vi "Configure Regulation Speed.vi"(8 "error in (no error)":errorcluster, 10 "Regulation Speed (1: Medium)":u16(ring)=1 items=["Slow", "Medium", "Fast"], 11 "VISA resource name":refnum<visa-resource-name>) -> (0 "error out":errorcluster, 3 "VISA resource name out":refnum<visa-resource-name>)   [LabVIEW 2017, in "HH PLI Series.lvlib"]
doc: "Sets the regulation speed of the instrument controller."
uses:
  HH PLI Series.lvlib
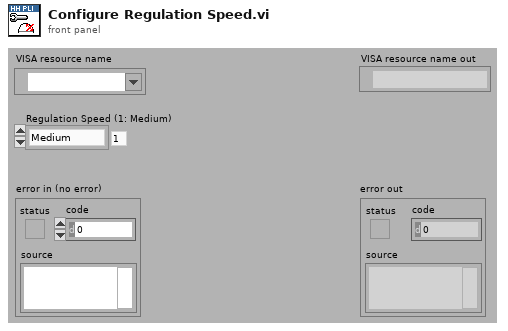
[diagram p1: front panel]
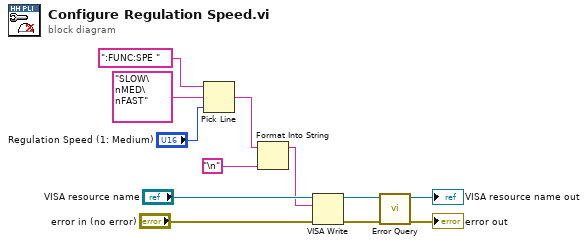
[diagram p0: block diagram]
diagram:
  n1 = Pick Line(string ("")=":FUNC:SPE ", multi-line string="SLOW\nMED\nFAST", line index="Regulation Speed (1: Medium)") -> (output string=w2:string)
  n2 = Format Into String(initial string=w2, "\n") -> (resulting string=w1:string)  [unwired: 2 in, 1 out]
  n3 = VISA Write(VISA resource name="VISA resource name", write buffer=w1, error in (no error)="error in (no error)") -> (VISA resource name out=w11:refnum<visa-resource-name>, error out=w10:errorcluster)  [unwired: 1 out]
  n4 = call "Error Query.vi"("error in (no error)"=w10, "VISA resource name"=w11) -> ("error out"=→"error out":errorcluster, "VISA resource name out"=→"VISA resource name out":refnum<visa-resource-name>)  [unwired: 6 in, 2 out]
